vi "MathCad_Matrix_Set_1D.vi"(3 "error in":errorcluster, 4 "1D Array":dbl[](array[numeric]) format="%.2f", 5 "Mathcad.IMatrixValue Refnum in":refnum<k7>, 6 "Worksheet Reference In":refnum<k7>) -> (0 "error out":errorcluster, 1 "Mathcad.IMatrixValue Refnum out":refnum<k7>, 2 "Worksheet Reference Out":refnum<k7>)   [LabVIEW 2015]
doc: "Sets the value of the reference. This must be done before inserting into a worksheet."
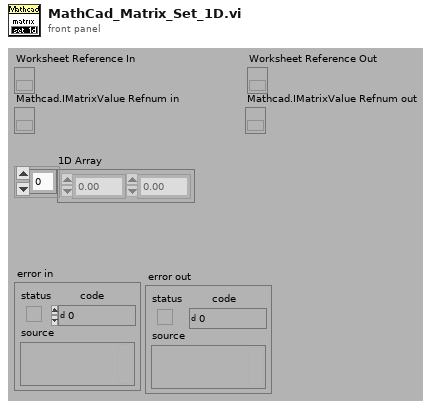
[diagram p1: front panel]
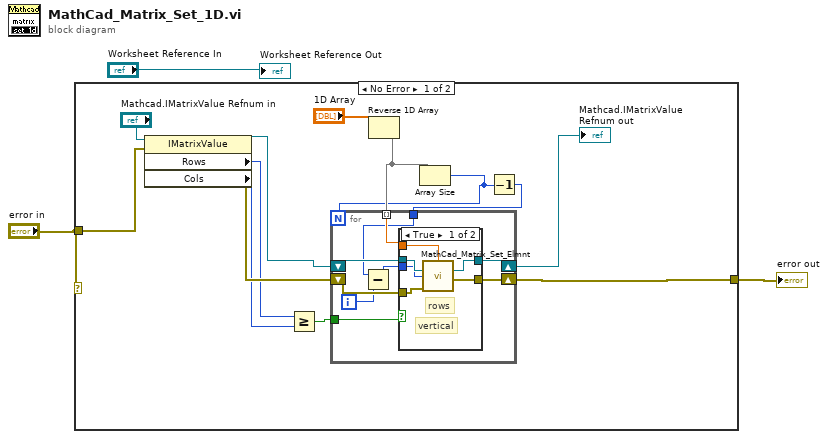
[diagram p0: block diagram]
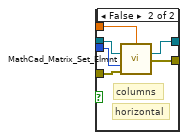
[diagram p2: hidden frame]
diagram:
  n1 = case shown="No Error" "error in" {
    tunnel: [w15 w38] -> w2
    tunnel: "error in" -> [w12 w38]
    frame No Error {
      n2 = property class="IMatrixValue"(reference="Mathcad.IMatrixValue Refnum in", error in=w12) -> (reference out=w14:refnum<k7>, error out=w11:errorcluster, "Rows"=w10:i32, "Cols"=w9:i32)
      n3 = Greater Or Equal?(x=w10, y=w9) -> (x >= y?=w8:bool)
      n4 = Reverse 1D Array(array="1D Array") -> (reversed array=w6:dbl[])
      n5 = Array Size(array=w6) -> (size(s)=w5:i32)
      n6 = Decrement(x=w5) -> (x-1=w4:i32)
      n7 = for {
        N: w5 -> [_]
        shift-right: [w25] -> w16
        shift-left: w14 -> [w24]
        shift-right: [w23] -> w15
        shift-left: w11 -> [w22]
        tunnel: w6 -> [w21] mode=indexing
        tunnel: w8 -> [w20]
        tunnel: w4 -> [w19]
        i -> [w17]
        n8 = Subtract(x=w19, y=w17) -> (x-y=w18:i32)
        n9 = case shown="True" w20 {
          tunnel: [w31 w37] -> w25
          tunnel: w24 -> [w30 w36]
          tunnel: [w29 w35] -> w23
          tunnel: w22 -> [w28 w34]
          tunnel: w21 -> [w26 w33]
          tunnel: w18 -> [w27 w32]
          frame True {
            # "vertical"
            # "rows"
            n10 = call "MathCad_Matrix_Set_Elmnt.vi"("value"=w26, "Mathcad.IMatrixValue"=w30, "row"=w27, "error in"=w28) -> ("Mathcad.IMatrixValue Refnum out"=w31:refnum<k7>, "error out"=w29:errorcluster)  [unwired: 9 in, 1 out]
          }
          frame False {
            # "horizontal"
            # "columns"
            n11 = call "MathCad_Matrix_Set_Elmnt.vi"("value"=w33, "Mathcad.IMatrixValue"=w36, "col"=w32, "error in"=w34) -> ("Mathcad.IMatrixValue Refnum out"=w37:refnum<k7>, "error out"=w35:errorcluster)  [unwired: 9 in, 1 out]
          }
        }
      }
      "Mathcad.IMatrixValue Refnum out" <- w16
    }
    frame Error {
    }
  }
  "error out" <- w2
  "Worksheet Reference Out" <- "Worksheet Reference In"
